vi "DAQ_PS Initialize.vi"(0 "Physical channels":tag="TS1Mod1/power", 11 "error in":errorcluster) -> (4 "DAQmx Task Out":refnum<k21>, 15 "error out":errorcluster)   [LabVIEW 2021, in "DAQ_Power Supply Source and Measure.lvlib"]
doc: "Initialize power supply channels to source power"
uses:
  DAQ_Power Supply Source and Measure.lvlib
  <vilib>/DAQmx/create/channels.llb/DAQmx Create Channel (Power).vi
panel:
  # "Inputs"
  # "Outputs"
  # "Overview:\nThis VI initializes power supply and provides the DAQmx Task Out\n\nHardware Requirement:  TS-15200\n\nSoftware Requirement: NI DAQmx 22Q4 or later\n\n\nInstructions:\n\t1. Input the physical channel on which power supply source and measurements are taken in Physical channel control.\n2. Get the power supply task from DAQmx Task Out which stores the reference to the virtual power supply channels.\nNote: User can use the DAQmx Task on other VI in this library to configure and initiate power supply source and measurements."
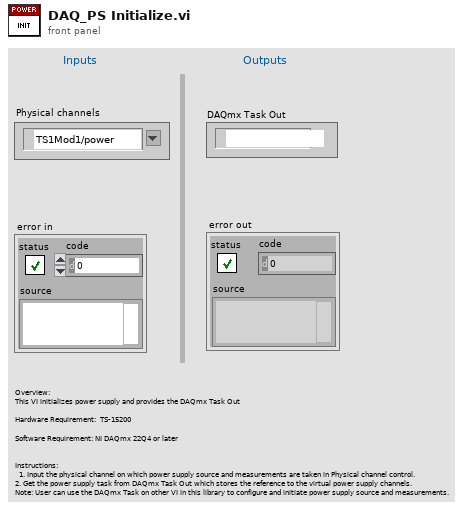
[diagram p1: front panel]
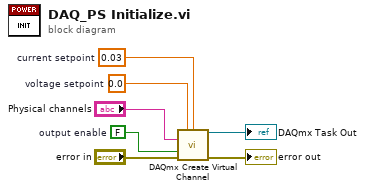
[diagram p0: block diagram]
diagram:
  w6 = FALSE  # output enable
  w1 = 0.03  # current setpoint
  w2 = 0.0  # voltage setpoint
  n1 = call-poly <vilib>:"DAQmx Create Virtual Channel.vi"("voltage setpoint"=w2, "current setpoint"=w1, "physical channels"="Physical channels", "output enable"=w6, "error in"="error in") -> ("task out"=→"DAQmx Task Out":refnum<k21>, "error out"=→"error out":errorcluster)  [unwired: 9 in]
